vi "RecordNoiseDifference.vi"(3 "All":dbl, 4 "All f":dbl, 5 "Blue f":dbl, 6 "Green  f":dbl, 7 "Red f":dbl, 8 "Blue":dbl, 9 "Green":dbl, 10 "file path (use dialog)":path, 11 "Red":dbl) -> ()   [LabVIEW 2016]
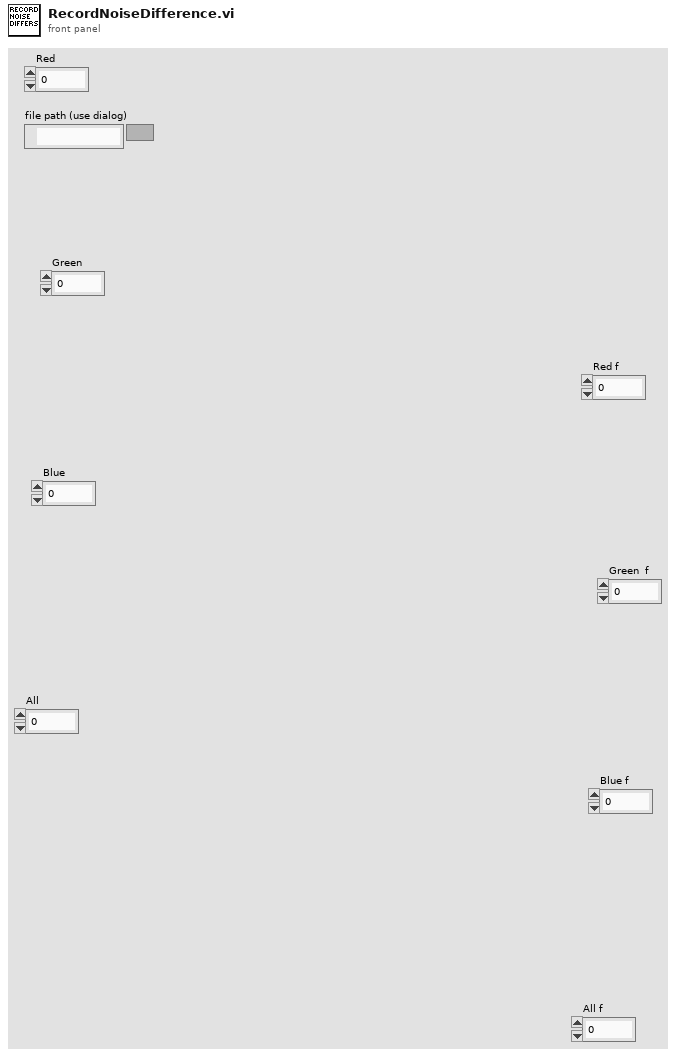
[diagram p1: front panel]
types:
  T1 = enum16{"open", "replace", "create", "open or create", "replace or create", "replace or create with confirmation"}
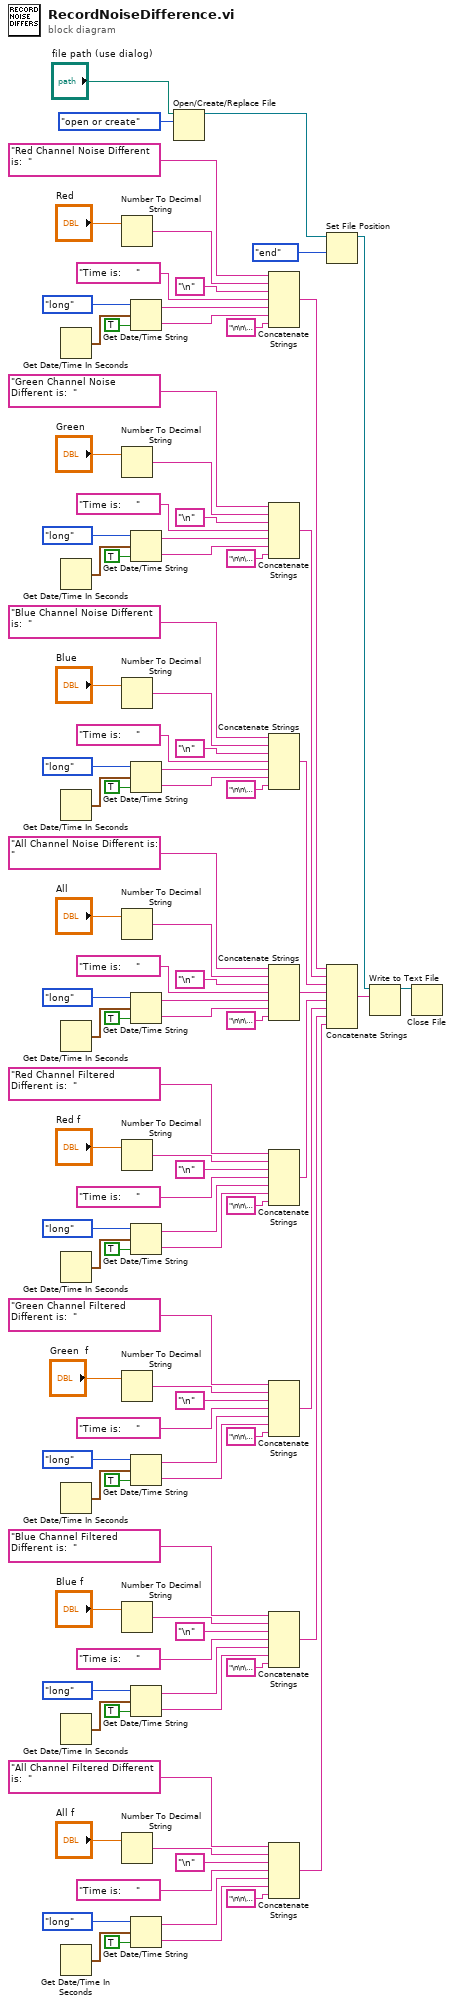
[diagram p0: block diagram]
diagram:
  n1 = Get Date/Time In Seconds() -> (seconds since 1Jan1904=w96:timestamp)
  n2 = Get Date/Time In Seconds() -> (seconds since 1Jan1904=w78:timestamp)
  n3 = Get Date/Time In Seconds() -> (seconds since 1Jan1904=w73:timestamp)
  n4 = Get Date/Time In Seconds() -> (seconds since 1Jan1904=w52:timestamp)
  n5 = Get Date/Time In Seconds() -> (seconds since 1Jan1904=w8:timestamp)
  n6 = Get Date/Time In Seconds() -> (seconds since 1Jan1904=w24:timestamp)
  n7 = Get Date/Time In Seconds() -> (seconds since 1Jan1904=w29:timestamp)
  n8 = Get Date/Time In Seconds() -> (seconds since 1Jan1904=w46:timestamp)
  n9 = Number To Decimal String(number="Red") -> (decimal integer string=w88:string)  [unwired: 1 in]
  n10 = Number To Decimal String(number="Green") -> (decimal integer string=w85:string)  [unwired: 1 in]
  n11 = Number To Decimal String(number="Blue") -> (decimal integer string=w66:string)  [unwired: 1 in]
  n12 = Number To Decimal String(number="All") -> (decimal integer string=w59:string)  [unwired: 1 in]
  n13 = Number To Decimal String(number="Red f") -> (decimal integer string=w15:string)  [unwired: 1 in]
  n14 = Number To Decimal String(number="Green  f") -> (decimal integer string=w17:string)  [unwired: 1 in]
  n15 = Number To Decimal String(number="Blue f") -> (decimal integer string=w36:string)  [unwired: 1 in]
  n16 = Number To Decimal String(number="All f") -> (decimal integer string=w39:string)  [unwired: 1 in]
  n17 = Get Date/Time String(date format (0)=enum16{"short", "long", "abbreviated"}."long", seconds (now)=w96, want seconds? (F)=TRUE) -> (date string=w92:string, time string=w91:string)
  n18 = Get Date/Time String(date format (0)=enum16{"short", "long", "abbreviated"}."long", seconds (now)=w78, want seconds? (F)=TRUE) -> (date string=w82:string, time string=w83:string)
  n19 = Get Date/Time String(date format (0)=enum16{"short", "long", "abbreviated"}."long", seconds (now)=w73, want seconds? (F)=TRUE) -> (date string=w69:string, time string=w68:string)
  n20 = Get Date/Time String(date format (0)=enum16{"short", "long", "abbreviated"}."long", seconds (now)=w52, want seconds? (F)=TRUE) -> (date string=w56:string, time string=w57:string)
  n21 = Get Date/Time String(date format (0)=enum16{"short", "long", "abbreviated"}."long", seconds (now)=w8, want seconds? (F)=TRUE) -> (date string=w12:string, time string=w13:string)
  n22 = Get Date/Time String(date format (0)=enum16{"short", "long", "abbreviated"}."long", seconds (now)=w24, want seconds? (F)=TRUE) -> (date string=w20:string, time string=w19:string)
  n23 = Get Date/Time String(date format (0)=enum16{"short", "long", "abbreviated"}."long", seconds (now)=w29, want seconds? (F)=TRUE) -> (date string=w33:string, time string=w34:string)
  n24 = Get Date/Time String(date format (0)=enum16{"short", "long", "abbreviated"}."long", seconds (now)=w46, want seconds? (F)=TRUE) -> (date string=w42:string, time string=w41:string)
  n25 = Open/Create/Replace File(file path (use dialog)="file path (use dialog)", operation (0:open)=T1."open or create") -> (refnum out=w99:refnum<file>)  [unwired: 4 in, 2 out]
  n26 = Concatenate Strings("Red Channel Noise Different is:  ", w88, "\n", "Time is:     ", w92, w91, "\n\n\n\n") -> (w64:string)
  n27 = Concatenate Strings("Green Channel Noise Different is:  ", w85, "\n", "Time is:     ", w82, w83, "\n\n\n\n") -> (w63:string)
  n28 = Concatenate Strings("Blue Channel Noise Different is:  ", w66, "\n", "Time is:     ", w69, w68, "\n\n\n\n") -> (w62:string)
  n29 = Concatenate Strings("All Channel Noise Different is:  ", w59, "\n", "Time is:     ", w56, w57, "\n\n\n\n") -> (w49:string)
  n30 = Concatenate Strings("Red Channel Filtered Different is:  ", w15, "\n", "Time is:     ", w12, w13, "\n\n\n\n") -> (w4:string)
  n31 = Concatenate Strings("Green Channel Filtered Different is:  ", w17, "\n", "Time is:     ", w20, w19, "\n\n\n\n") -> (w3:string)
  n32 = Concatenate Strings("Blue Channel Filtered Different is:  ", w36, "\n", "Time is:     ", w33, w34, "\n\n\n\n") -> (w2:string)
  n33 = Concatenate Strings("All Channel Filtered Different is:  ", w39, "\n", "Time is:     ", w42, w41, "\n\n\n\n") -> (w1:string)
  n34 = Set File Position(refnum=w99, from (0:start)=enum16{"start", "end", "current"}."end") -> (refnum out=w98:refnum<file>)  [unwired: 2 in, 1 out]
  n35 = Concatenate Strings(w64, w63, w62, w49, w4, w3, w2, w1) -> (w61:string)
  n36 = Write to Text File(file (use dialog)=w98, text=w61) -> (refnum out=w97:refnum<file>)  [unwired: 2 in, 2 out]
  n37 = Close File(refnum=w97) -> ()  [unwired: 1 in, 2 out]
